vi "RemoveOldBusNumber.vi"(8 "ErrorArray In":errorcluster[](array[cluster]), 11 "clFrontPanelControlRefs In":T1) -> (0 "ErrorArray Out":errorcluster[](array[cluster]), 3 "clFrontPanelControlRefs Out":T1)   [LabVIEW 2014, in "TestFramework.lvlib"]
uses:
  TestFramework.lvlib
  TypeDefs/clFrontPanelControlRefs.ctl
  FGenPlugins/MyPluginBaseClass/TypeDef/PluginParams.ctl
  WfrmGenerator/WfrmPlugins/EventPluginBaseClass/TypeDefs/dblEvtSignalArray.ctl
  FGenPlugins/MyPluginBaseClass/TypeDef/CreateArbWfrmParams.ctl
  WfrmGenerator/WfrmPlugins/EventPluginBaseClass/TypeDefs/clEvtConfig.ctl
  WfrmGenerator/WfrmModule/PublicAPI/Arguments/Requests/dblEvtParams.ctl
  FGenPlugins/MyPluginBaseClass/TypeDef/ConfigArbWfrmParams.ctl
  FGenPlugins/MyPluginBaseClass/TypeDef/TriggerParams.ctl
  <userlib>/NIST/NISTErrorLib/NISTErrorLib.lvlib
  FGenPlugins/MyPluginBaseClass/NISTFGenPluginsBase.lvclass
  WfrmGenerator/WfrmPlugins/EventPluginBaseClass/BaseWfrmPlugin.lvclass
  WfrmGenerator/WfrmModule/WfrmModule.lvlib
panel:
  # "When you add a control \non the front panel, add a\nreference for it in this\ntype def.  This cluster\nwill hold all of the refer-\nences to the front panel\ncontrols in order to pass\nthese control references \nto subvis."
  # "When you add a control \non the front panel, add a\nreference for it in this\ntype def.  This cluster\nwill hold all of the refer-\nences to the front panel\ncontrols in order to pass\nthese control references \nto subvis."
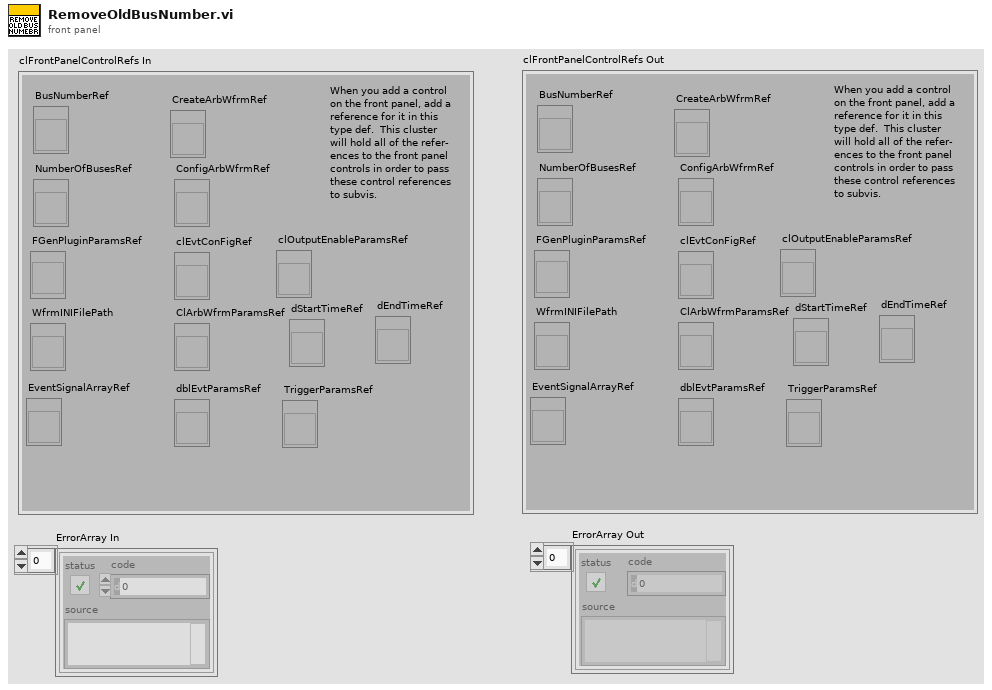
[diagram p1: front panel]
types:
  T1 = typedef "TestFramework.lvlib/clFrontPanelControlRefs.ctl" = cluster{"BusNumberRef":refnum<vi>, "NumberOfBusesRef":refnum<vi>, "FGenPluginParamsRef":refnum<vi>, "WfrmINIFilePath":refnum<vi>, "EventSignalArrayRef":refnum<vi>, "CreateArbWfrmRef":refnum<vi>, "clEvtConFigRef":refnum<vi>, "dblEvtParamsRef":refnum<vi>, "clOutputEnableParamsRef":refnum<vi>, "ConfigArbWfrmRef":refnum<vi>, "ClArbWfrmParamsRef":refnum<vi>, "dStartTimeRef":refnum<vi>, "dEndTimeRef":refnum<vi>, "TriggerParamsRef":refnum<vi>}
  T2 = typedef "LVStringsAndValuesArrayTypeDef_U8.ctl" = cluster{"String":string, "Value":u8}[]
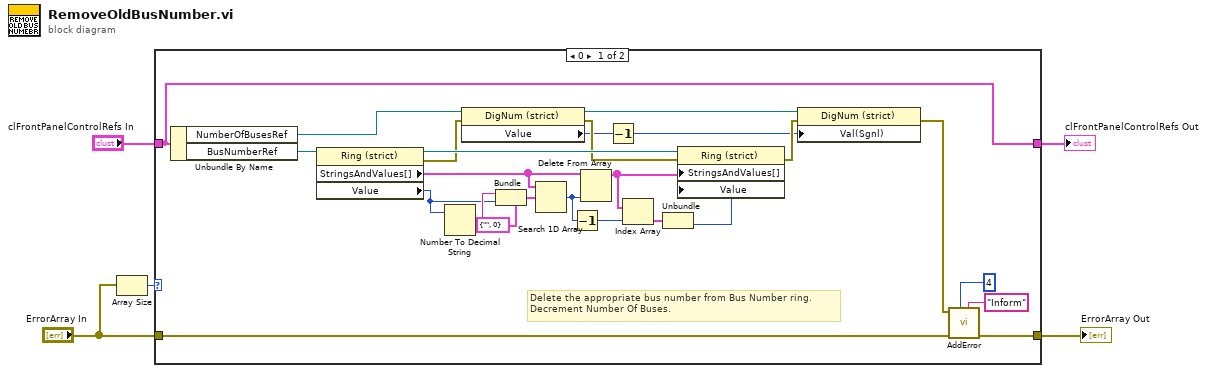
[diagram p0: block diagram]
diagram:
  n1 = Array Size(array="ErrorArray In") -> (size(s)=w5:i32)
  n2 = case shown="0" w5 {
    tunnel: "clFrontPanelControlRefs In" -> [w19 w32]
    tunnel: "ErrorArray In" -> [w21 w31]
    tunnel: [w20 w31] -> w2
    tunnel: [w19 w32] -> w1
    frame 0 {
      # "Delete the appropriate bus number from Bus Number ring.\nDecrement Number Of Buses."
      n3 = Unbundle By Name(w19) -> ("NumberOfBusesRef"=w16:refnum<vi>, "BusNumberRef"=w30:refnum<vi>)
      n4 = property class="Ring (strict)"(reference=w30) -> (reference out=w26:refnum<vi>, error out=w17:errorcluster, "StringsAndValues[]"=w11:T2, "Value"=w10:u8)  [unwired: 1 in]
      n5 = Number To Decimal String(number=w10) -> (decimal integer string=w28:string)  [unwired: 1 in]
      n6 = property class="DigNum (strict)"(reference=w16, error in=w17) -> (reference out=w14:refnum<vi>, error out=w18:errorcluster, "Value"=w15:u8)
      n7 = Bundle(cluster=cluster{"String":string, "Value":u8} {"String"="", "Value"=0} ("element"), "String"=w28, "Value"=w10) -> (w27:cluster{"String":string, "Value":u8})
      n8 = Search 1D Array(1D array=w11, element=w27) -> (index of element=w12:i32)  [unwired: 1 in]
      n9 = Decrement(x=w12) -> (x-1=w9:i32)
      n10 = Delete From Array(array=w11, index=w12) -> (array with subset deleted=w8:T2)  [unwired: 1 in, 1 out]
      n11 = Decrement(x=w15) -> (x-1=w13:u8)
      n12 = Index Array(array=w8, index=w9) -> (element=w7:cluster{"String":string, "Value":u8})
      n13 = Unbundle(w7) -> ("Value"=w6:u8)  [unwired: 1 out]
      n14 = property class="Ring (strict)"(reference=w26, error in=w18, "StringsAndValues[]"=w8, "Value"=w6) -> (error out=w25:errorcluster)  [unwired: 1 out]
      n15 = property class="DigNum (strict)"(reference=w14, error in=w25, "Val(Sgnl)"=w13) -> (error out=w22:errorcluster)  [unwired: 1 out]
      n16 = call <userlib>:"AddError.vi"("Severity"="Inform" ("String"), "Priority"=u8 4, "ErrorArray"=w21, "error in (no error)"=w22) -> ("ErrorArray"=w20:errorcluster[])  [unwired: 6 in, 1 out]
    }
    frame 1, Default {
    }
  }
  "clFrontPanelControlRefs Out" <- w1
  "ErrorArray Out" <- w2
